vi "Configure.vi"(8 "error in (no error)":errorcluster) -> (0 "error out":errorcluster, 1 "trend point registrations":T1[](array[typedef]), 3 "config":T3, 5 "valid config":bool)   [LabVIEW 2017, in "IrAnalysis.lvlib"]
uses:
  <vilib>/addons/InsightCM/Devices/Shared/Ir/IrAnalysis/IrAnalysis.lvlib
  <vilib>/addons/InsightCM/Devices/Shared/Ir/IrAnalysis/controls/config.ctl
  <vilib>/addons/InsightCM/Devices/Shared/Ir/IrAnalysis/controls/roi.ctl
  <vilib>/addons/InsightCM/Devices/Shared/Ir/IrAnalysis/controls/metric.ctl
  <vilib>/addons/InsightCM/MessageBus/Base/controls/MetricDefinitionInstance.ctl
  <vilib>/addons/InsightCM/MessageBus/Base/controls/KeyValuePair.ctl
  <vilib>/addons/InsightCM/Devices/Shared/Common/DataEventCreator/controls/RegisterTrendPoints.ctl
  <vilib>/addons/InsightCM/Devices/Shared/Common/DataEventCreator/controls/Registry_Trend.ctl
  <vilib>/addons/InsightCM/Utilities/GlobalConfiguration/GlobalConfiguration.lvlib
  <vilib>/addons/InsightCM/Utilities/PropertyHelpers/PropertyHelpers.lvlib
  <vilib>/addons/InsightCM/Utilities/DeviceModelHelpers/DeviceModelHelpers.lvlib
  <vilib>/addons/InsightCM/Devices/Shared/Common/DataEventCreator/DataEventCreator.lvlib
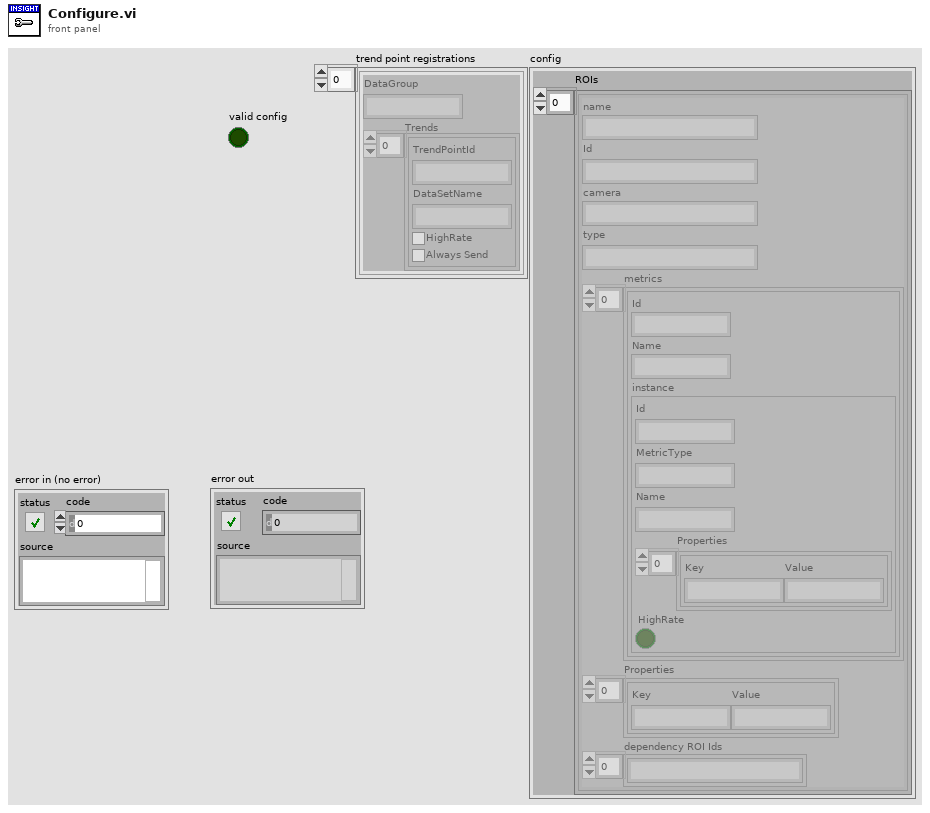
[diagram p1: front panel]
types:
  T1 = typedef "DataEventCreator.lvlib/RegisterTrendPoints.ctl" = cluster{"DataGroup":string, "Trends":T2[]}
  T2 = typedef "DataEventCreator.lvlib/Registry_Trend.ctl" = cluster{"TrendPointId":string, "DataSetName":string, "HighRate":bool, "Always Send":bool}
  T3 = typedef "IrAnalysis.lvlib/config.ctl" = cluster{"ROIs":T4[]}
  T4 = typedef "IrAnalysis.lvlib/roi.ctl" = cluster{"name":string, "Id":string, "camera":string, "type":string, "metrics":T5[], "Properties":T7[], "dependency ROI Ids":string[]}
  T5 = typedef "IrAnalysis.lvlib/metric.ctl" = cluster{"Id":string, "Name":string, "instance":T6}
  T6 = typedef "MetricDefinitionInstance.ctl" = cluster{"Id":string, "MetricType":string, "Name":string, "Properties":T7[], "HighRate":bool}
  T7 = typedef "KeyValuePair.ctl" = cluster{"Key":string, "Value":string}
  T8 = typedef "R2_DeviceModel.ctl" = cluster{"Device":T9, "Channels":T19[], "Tags":T21[]}
  T9 = typedef "R2_Device.ctl" = cluster{"Id":string, "Name":string, "DeviceType":string, "HardwareName":string, "IpAddress":string, "HardwareInfo":T7[], "ApplicationType":string, "ApplicationVersion":string, "EquipmentIds":string[], "ConfigurationVersion":string, "State":T10, "Properties":T7[], "DataGroups":T11[], "BurstModeTrigger":T15, "SensorGroups":T16[]}
  T10 = typedef "DeviceState.ctl" = cluster{"Disabled":bool}
  T11 = typedef "R2_DataGroup.ctl" = cluster{"Name":string, "OperatingStates":T12[], "Properties":T7[], "EquipmentIds":string[], "AssetNodeId":string}
  T12 = typedef "OperatingState.ctl" = cluster{"Name":string, "Properties":T7[], "Triggers":T13[]}
  T13 = typedef "Trigger.ctl" = cluster{"Type":string, "Expression":string, "Conditions":T14[]}
  T14 = typedef "Condition.ctl" = cluster{"Source":string, "Type":string, "Operator":string, "CompareTo":string, "DwellSeconds":dbl}
  T15 = typedef "BurstModeTrigger.ctl" = cluster{"Trigger":T13, "SampleRate":string, "AcquisitionLength":string}
  T16 = typedef "DeviceSensorGroup.ctl" = cluster{"EquipId":string, "SensorGroupId":string, "Endpoints":T17[]}
  T17 = typedef "Endpoint.ctl" = cluster{"Type":string, "Address":string, "Properties":T7[], "Channels":T18[]}
  T18 = typedef "WirelessChannel.ctl" = cluster{"ChannelNumber":i32, "AssetId":string}
  T19 = typedef "R2_Channel.ctl" = cluster{"Id":string, "DeviceId":string, "Name":string, "ChannelType":string, "HardwareKey":string, "HardwareChannel":string, "DataGroup":string, "Keywords":string[], "EquipmentIds":string[], "Properties":T7[], "Metrics":T20[], "AssetNodeId":string, "MeasType":string, "AssetName":string}
  T20 = typedef "Metric.ctl" = cluster{"Id":string, "Name":string, "Unit":string, "Properties":T7[], "MetricDefinitionInstanceId":string}
  T21 = typedef "Tag.ctl" = cluster{"Id":string, "Path":string, "Name":string, "Datatype":string, "Props":T7[], "Keywords":string[]}
  T22 = typedef "AssetNode.ctl" = cluster{"Id":string, "Type":string, "Name":string, "ParentIds":string[], "State":T23, "MeasType":string, "Properties":T7[], "SensorGroups":T24[], "OperatingStates":T12[], "Metrics":T20[], "TrendAlarmRules":T25[], "References":T28[]}
  T23 = typedef "AssetState.ctl" = cluster{"Disabled":bool}
  T24 = typedef "AssetNodeSensorGroup.ctl" = cluster{"Id":string, "Type":string, "SensorIds":string[], "Triggers":T13[], "Properties":T7[]}
  T25 = typedef "TrendAlarmRule.ctl" = cluster{"Id":string, "AssetNodeId":string, "TrendId":string, "Disabled":bool, "OperatingState":string, "Operator":string, "Hysteresis":dbl, "OnDelaySeconds":dbl, "OffDelaySeconds":dbl, "Levels":T26[], "Properties":T7[]}
  T26 = typedef "TrendAlarmLevel.ctl" = cluster{"Severity":i32, "CompareTo":dbl, "Actions":T27[]}
  T27 = typedef "AlarmAction.ctl" = cluster{"Type":string, "Props":T7[]}
  T28 = typedef "AssetNodeReference.ctl" = cluster{"NodeId":string, "Name":string}
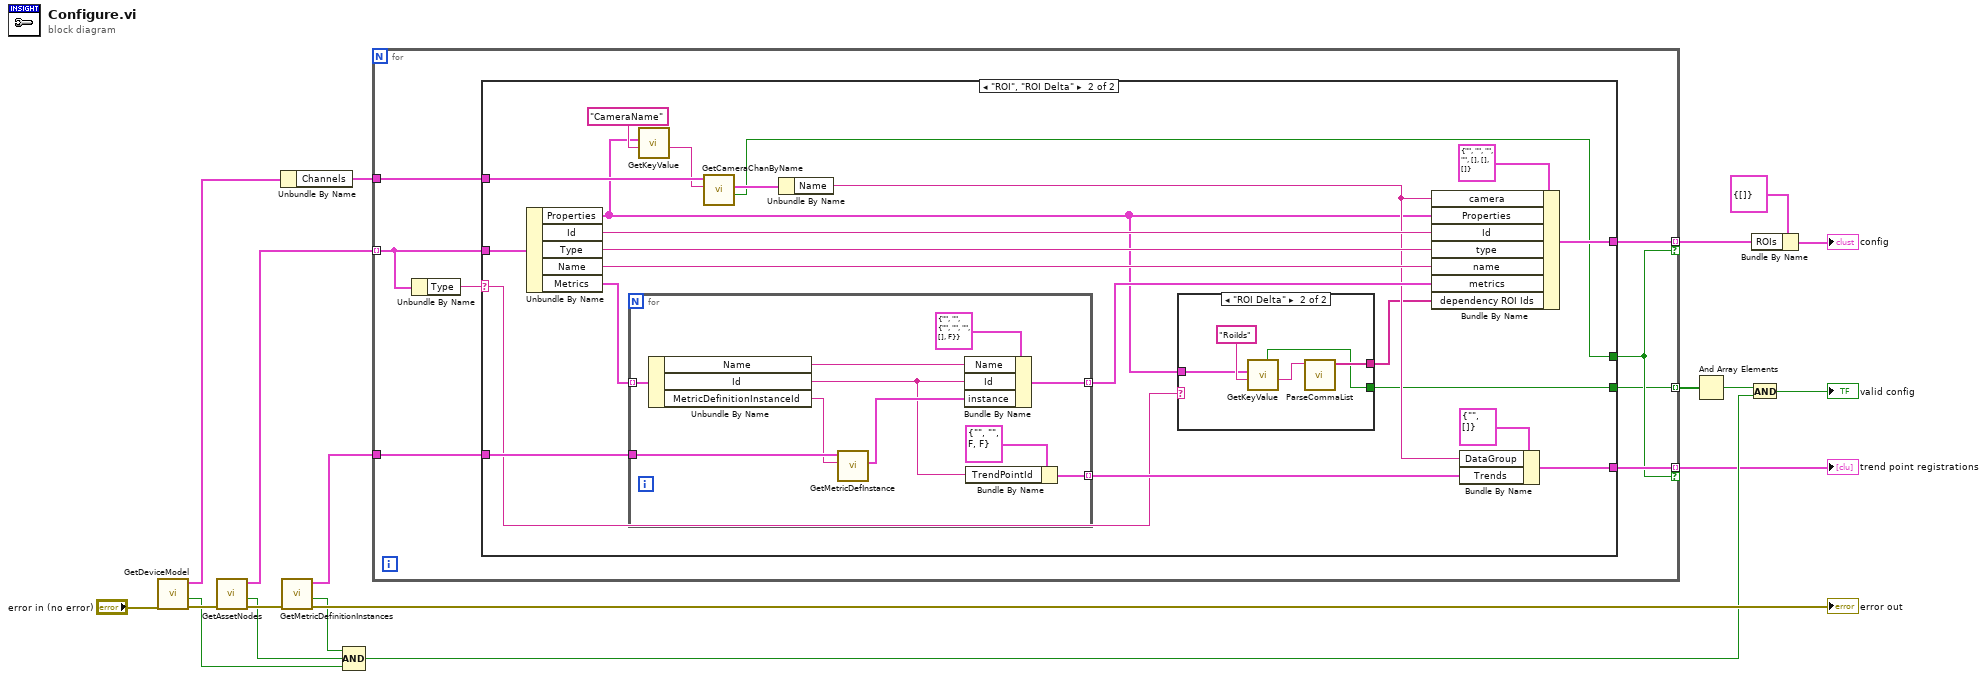
[diagram p0: block diagram]
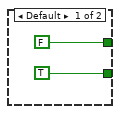
[diagram p2: hidden frame]
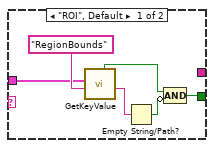
[diagram p3: hidden frame]
diagram:
  n1 = call <vilib>:"GetDeviceModel.vi"("error in (no error)"="error in (no error)") -> ("error out"=w15:errorcluster, "found"=w6:bool, "device model"=w18:T8)  [unwired: 8 in]
  n2 = call <vilib>:"GetAssetNodes.vi"("error in (no error)"=w15) -> ("error out"=w14:errorcluster, "found"=w7:bool, "AssetNodes"=w13:T22[])  [unwired: 8 in]
  n3 = Unbundle By Name(w18) -> ("Channels"=w12:T19[])
  n4 = call <vilib>:"GetMetricDefinitionInstances.vi"("error in (no error)"=w14) -> ("error out"=→"error out":errorcluster, "found"=w8:bool, "metrics"=w17:T6[])  [unwired: 8 in]
  n5 = Compound Arithmetic op=AND(w8, w7, w6) -> (w3:bool)
  n6 = for {
    tunnel: w17 -> [w27]
    tunnel: w13 -> [w24] mode=indexing
    tunnel: w12 -> [w25]
    tunnel: [w23] -> w11 mode=indexing if=w21
    tunnel: [w22] -> w1 mode=indexing if=w21
    tunnel: [w20] -> w5 mode=indexing
    n7 = Unbundle By Name(w24) -> ("Type"=w26:string)
    n8 = case shown="\"ROI\", \"ROI Delta\"" w26 {
      selector: w26 -> [_ w33]
      tunnel: w27 -> [_ w43]
      tunnel: w25 -> [_ w50]
      tunnel: w24 -> [_ w47]
      tunnel: [_ w41] -> w23
      tunnel: [_ w37] -> w22
      tunnel: [FALSE w30] -> w21
      tunnel: [TRUE ("found") w32] -> w20
      frame Default {
      }
      frame "ROI", "ROI Delta" {
        n9 = Unbundle By Name(w47) -> ("Properties"=w34:T7[], "Id"=w46:string, "Type"=w45:string, "Name"=w40:string, "Metrics"=w44:T20[])
        n10 = for {
          tunnel: w44 -> [w72] mode=indexing
          tunnel: w43 -> [w70]
          tunnel: [w67] -> w42 mode=indexing
          tunnel: [w65] -> w38 mode=indexing
          n11 = Unbundle By Name(w72) -> ("Name"=w64:string, "Id"=w66:string, "MetricDefinitionInstanceId"=w69:string)
          n12 = call <vilib>:"GetMetricDefInstance.vi"("metric definition instance id"=w69, "metric definition instances"=w70) -> ("metric definition instance"=w68:T6)  [unwired: 7 in, 2 out]
          n13 = Bundle By Name(cluster=T5 {"Id"="", "Name"="", "instance"={"Id"="", "MetricType"="", "Name"="", "Properties"=[], "HighRate"=FALSE}} ("metric"), "Name"=w64, "Id"=w66, "instance"=w68) -> (w67:T5)
          n14 = Bundle By Name(cluster=T2 {"TrendPointId"="", "DataSetName"="", "HighRate"=FALSE, "Always Send"=FALSE} ("Trend"), "TrendPointId"=w66) -> (w65:T2)
        }
        n15 = call <vilib>:"GetKeyValue.vi"("key"="CameraName", "key value pairs"=w34) -> ("value"=w49:string)  [unwired: 7 in, 2 out]
        n16 = call <vilib>:"GetCameraChanByName.vi"("camera name"=w49, "channels"=w50) -> ("found"=w30:bool, "channel (camera)"=w39:T19)  [unwired: 7 in, 1 out]
        n17 = Unbundle By Name(w39) -> ("Name"=w36:string)
        n18 = case shown="\"ROI Delta\"" w33 {
          tunnel: [_ w61] -> w35
          tunnel: w34 -> [w56 w59]
          tunnel: [w54 w58] -> w32
          frame "ROI", Default {
            n19 = call <vilib>:"GetKeyValue.vi"("key"="RegionBounds", "key value pairs"=w56) -> ("value"=w55:string, "found"=w53:bool)  [unwired: 7 in, 1 out]
            n20 = Empty String/Path?(string/path=w55) -> (empty?=w52:bool)
            n21 = Compound Arithmetic op=AND(w53, invert w52) -> (w54:bool)
          }
          frame "ROI Delta" {
            n22 = call <vilib>:"GetKeyValue.vi"("key"="RoiIds", "key value pairs"=w59) -> ("value"=w60:string, "found"=w58:bool)  [unwired: 7 in, 1 out]
            n23 = call <vilib>:"ParseCommaList.vi"("value"=w60) -> ("Array"=w61:string[])  [unwired: 10 in]
          }
        }
        n24 = Bundle By Name(cluster=T4 {"name"="", "Id"="", "camera"="", "type"="", "metrics"=[], "Properties"=[], "dependency ROI Ids"=[]} ("roi"), "camera"=w36, "Properties"=w34, "Id"=w46, "type"=w45, "name"=w40, "metrics"=w42, "dependency ROI Ids"=w35) -> (w41:T4)
        n25 = Bundle By Name(cluster=T1 {"DataGroup"="", "Trends"=[]} ("RegisterTrend"), "DataGroup"=w36, "Trends"=w38) -> (w37:T1)
      }
    }
  }
  "trend point registrations" <- w1
  n26 = And Array Elements(Boolean array=w5) -> (logical AND=w4:bool)
  n27 = And(x=w4, y=w3) -> (x .and. y?=→"valid config":bool)
  n28 = Bundle By Name(cluster=T3 {"ROIs"=[]} ("config"), "ROIs"=w11) -> (→"config":T3)
